vi "EventBuilder.publish description service.vi"(0 "i ref in":refnum<vi>, 1 "myHeaderData":T1, 2 "DAQDevices":string[](array[string]), 3 "ms timeout (10000)":i32=10000, 5 "error in (no error)":errorcluster) -> (14 "i ref out":refnum<vi>, 17 "timed out":bool, 19 "error out":errorcluster)   [LabVIEW 2014, in "EventBuilder.lvlib"]
doc: "Publishes the service \"EVENTBUILDERNAME_dataDescription\" and stores the data into the attribute data. Moreover, the eventID is reset to \"-1\".\n\nIf the service does not exist, it will be created. If the service data changes its size, the service is destroyed and recreated."
uses:
  EventBuilder.lvlib
  CS_Core/CSSystem/CoreDefs/CoreDefs.rawDataType.ctl
  CSlibraries-extern/DimLVEvent/LVDimInterface/LVDimInterface.lvlib
  CS_Core/CSSystem/CSSystemLib/CSSystemLib.lvlib
  CS_Core/CSSystem/CoreLib/CoreLib.lvlib
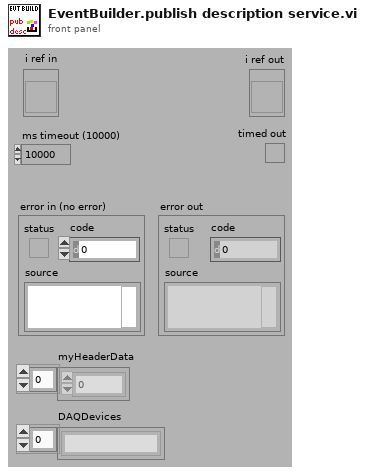
[diagram p1: front panel]
types:
  T1 = typedef "CoreDefs.rawDataType.ctl" = i8[]
  T2 = typedef "EventBuilder.lvlib/EventBuilder.i attribute.ctl" = cluster{"header":string, "DAQObjs":string[], "headerID":dbl, "eventID":i32, "dataDescriptionID":i32, "eventDataID":i32, "eventDataSize":i32, "dataDescriptionSize":i32}
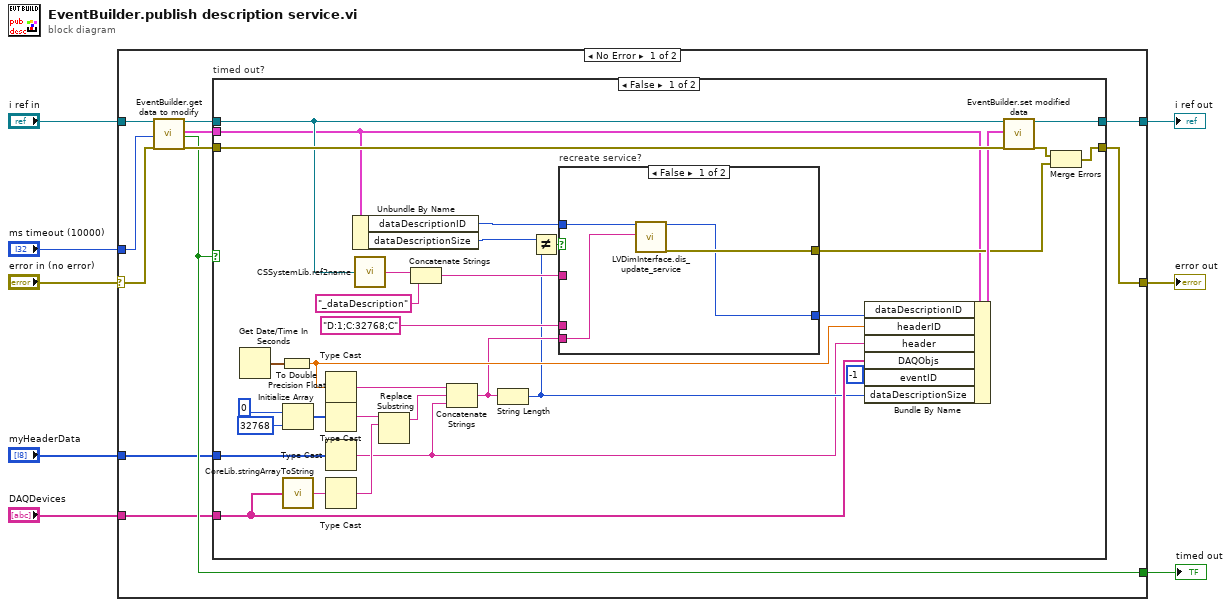
[diagram p0: block diagram]
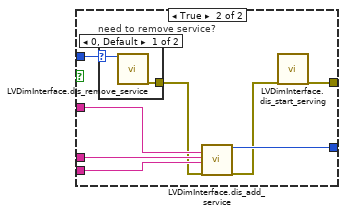
[diagram p2: hidden frame]
diagram:
  n1 = case shown="No Error" "error in (no error)" {
    selector: "error in (no error)" -> [w11 w68]
    tunnel: "i ref in" -> [w19 w69]
    tunnel: [w18 w68] -> w7
    tunnel: [w17 w69] -> w6
    tunnel: "ms timeout (10000)" -> [w13 _]
    tunnel: [w12 _] -> w4
    tunnel: "myHeaderData" -> [w10 _]
    tunnel: "DAQDevices" -> [w9 _]
    frame No Error {
      n2 = call "EventBuilder.get data to modify.vi"("i ref in"=w19, "ms timeout (10000)"=w13, "error in (no error)"=w11) -> ("i ref out"=w16:refnum<vi>, "i attribute"=w14:T2, "timed out"=w12:bool, "error out"=w15:errorcluster)  [unwired: 13 in]
      n3 = case "timed out?" shown="False" w12 {
        tunnel: [w33 w66] -> w18
        tunnel: [w51 w67] -> w17
        tunnel: w16 -> [w49 w67]
        tunnel: w15 -> [w50 w66]
        tunnel: w14 -> [w28 _]
        tunnel: w10 -> [w22 _]
        tunnel: w9 -> [w31 _]
        frame False {
          n4 = Get Date/Time In Seconds() -> (seconds since 1Jan1904=w44:timestamp)
          n5 = To Double Precision Float(number=w44) -> (double precision float=w30:dbl)
          n6 = Initialize Array(i8 0, 32768 ("dimension size")) -> (w41:i8[])
          n7 = call "CoreLib.stringArrayToString.vi"("Array"=w31) -> ("String"=w39:string)
          n8 = Type Cast(x=w30) -> (*(type *) &x=w38:string)  [unwired: 1 in]
          n9 = Type Cast(x=w41) -> (*(type *) &x=w40:string)  [unwired: 1 in]
          n10 = Type Cast(x=w22) -> (*(type *) &x=w20:string)  [unwired: 1 in]
          n11 = Type Cast(x=w39) -> (*(type *) &x=w21:string)  [unwired: 1 in]
          n12 = Unbundle By Name(w28) -> ("dataDescriptionID"=w24:i32, "dataDescriptionSize"=w26:i32)
          n13 = call "CSSystemLib.ref2name.vi"("obj refnum"=w49) -> ("name"=w48:string)
          n14 = Replace Substring(4:w21, 5:w40) -> (1:w37:string)  [unwired: 2 in, 1 out]
          n15 = Concatenate Strings(w48, "_dataDescription" ("string")) -> (w46:string)
          n16 = Concatenate Strings(w38, w37, w20) -> (w27:string)
          n17 = String Length(string=w27) -> (length=w23:i32)
          n18 = Not Equal?(x=w26, y=w23) -> (x != y?=w25:bool)
          n19 = case "recreate service?" shown="False" w25 {
            tunnel: w46 -> [_ w63]
            tunnel: "D:1;C:32768;C" ("typeDescriptor") -> [_ w62]
            tunnel: [w53 w61] -> w36
            tunnel: [w54 w57] -> w32
            tunnel: w27 -> [w52 w60]
            tunnel: w24 -> [w55 w59]
            frame False {
              n20 = call "LVDimInterface.dis_update_service.vi"("my_serviceID"=w55, "data"=w52) -> ("my_serviceID out"=w53:i32, "error out"=w54:errorcluster)  [unwired: 15 in, 1 out]
            }
            frame True {
              n21 = case "need to remove service?" shown="0, Default" w59 {
                selector: w59 -> [w65 _]
                tunnel: [w64 _] -> w58
                frame 0, Default {
                  n22 = call "LVDimInterface.dis_remove_service.vi"("my_serviceID"=w65) -> ("error out"=w64:errorcluster)  [unwired: 18 in]
                }
                frame -1 {
                }
              }
              n23 = call "LVDimInterface.dis_add_service.vi"("serviceName"=w63, "typeDescriptor"=w62, "data"=w60, "error in (no error)"=w58) -> ("my_serviceID"=w61:i32, "error out"=w56:errorcluster)  [unwired: 14 in]
              n24 = call "LVDimInterface.dis_start_serving.vi"("error in (no error)"=w56) -> ("error out"=w57:errorcluster)  [unwired: 17 in, 1 out]
            }
          }
          n25 = Bundle By Name(cluster=w28, "dataDescriptionID"=w36, "headerID"=w30, "header"=w20, "DAQObjs"=w31, "eventID"=-1, "dataDescriptionSize"=w23) -> (w35:T2)
          n26 = call "EventBuilder.set modified data.vi"("i ref in"=w49, "i attribute"=w35, "error in (no error)"=w50) -> ("i ref out"=w51:refnum<vi>, "error out"=w34:errorcluster)  [unwired: 15 in]
          n27 = Merge Errors(w34, w32) -> (w33:errorcluster)
        }
        frame True {
        }
      }
    }
    frame Error {
    }
  }
  "error out" <- w7
  "i ref out" <- w6
  "timed out" <- w4
